vi "UItoDAQconfig.vi"(8 "SamplingInfo":cluster{"Fs":dbl, "#S":i32}={"Fs"=1000.0, "#S"=1000}, 9 "AO Configuration":T7, 10 "AI Configuration":T10, 11 "DAQ_Manager.setDAQConfig":T1 {"DAQmx.AI.config"."input terminal configuration" items=["default"=-1, "RSE"=10083, "NRSE"=10078, "Differential"=10106, "Pseudodifferential"=12529]; "DAQmx.AI.config"."AI.Coupling" items=["AC"=10045, "DC"=10050, "GND"=10066]; "DAQmx.AO.config"."output terminal configuration" items=["Default"=-1, "RSE"=10083, "Differential"=10106, "Pseudodifferential"=12529]}) -> (3 "DAQ_Manager.setDAQConfig":T1 {"DAQmx.AI.config"."input terminal configuration" items=["default"=-1, "RSE"=10083, "NRSE"=10078, "Differential"=10106, "Pseudodifferential"=12529]; "DAQmx.AI.config"."AI.Coupling" items=["AC"=10045, "DC"=10050, "GND"=10066]; "DAQmx.AO.config"."output terminal configuration" items=["Default"=-1, "RSE"=10083, "Differential"=10106, "Pseudodifferential"=12529]})   [LabVIEW 2019, in "UI.Lockin.DAQ_config.lvclass"]
uses:
  UI.Lockin.DAQ_config.lvclass
  Typedefs/AI.config-array.ctl
  Typedefs/AI.config-cluster.ctl
  Typedefs/AI.coupling-enum.ctl
  Typedefs/446xAI-enum.ctl
  Typedefs/AO.config-array.ctl
  Typedefs/AO.config-cluster.ctl
  Typedefs/446xAO-enum.ctl
  DAQ_Manager/Typedefs/PrivateEvents--DAQ_Manager.setDAQConfig.ctl
  DAQmx.AI/Typedefs/DAQmx.AI_Config.ctl
  DAQmx.AI/Typedefs/AI.Coupling-enum.ctl
  DAQmx.AI/Typedefs/AI.Terminal-enum.ctl
  DAQmx.AO/Typedefs/DAQmx.AO_Config.ctl
  DAQmx.AO/Typedefs/AO.Terminal-enum.ctl
  DAQmx.AI/DAQmx.AI.lvclass
  DAQmx.AO/DAQmx.AO.lvclass
  DAQ_Manager/DAQ_Manager.lvclass
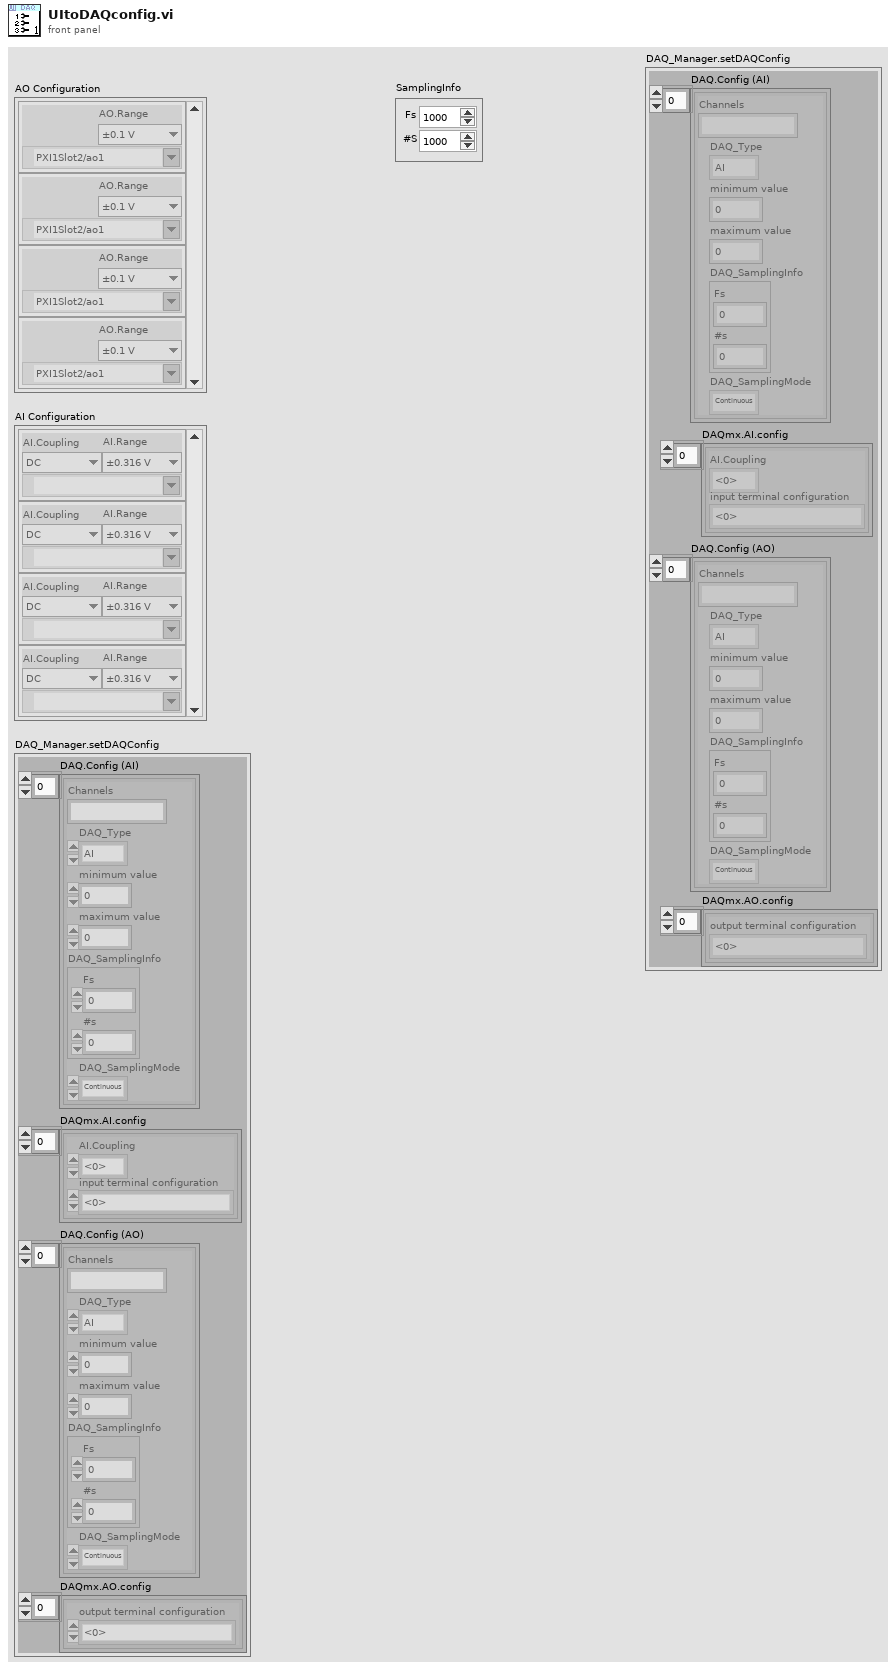
[diagram p1: front panel]
types:
  T1 = typedef "DAQ_Manager.lvclass/PrivateEvents--DAQ_Manager.setDAQConfig.ctl" = cluster{"DAQ.Config (AI)":cluster{"Channels":string, "DAQ_Type":enum16{"AI", "AO"}, "minimum value":dbl, "maximum value":dbl, "DAQ_SamplingInfo":cluster{"Fs":dbl, "#s":i32}, "DAQ_SamplingMode":enum16{"Continuous", "Finite"}}[], "DAQmx.AI.config":T2[], "DAQ.Config (AO)":cluster{"Channels":string, "DAQ_Type":enum16{"AI", "AO"}, "minimum value":dbl, "maximum value":dbl, "DAQ_SamplingInfo":cluster{"Fs":dbl, "#s":i32}, "DAQ_SamplingMode":enum16{"Continuous", "Finite"}}[], "DAQmx.AO.config":T5[]}
  T2 = typedef "DAQmx.AI.lvclass/DAQmx.AI_Config.ctl" = cluster{"AI.Coupling":T3, "input terminal configuration ":T4}
  T3 = typedef "DAQmx.AI.lvclass/AI.Coupling-enum.ctl" = i32
  T4 = typedef "DAQmx.AI.lvclass/AI.Terminal-enum.ctl" = i32
  T5 = typedef "DAQmx.AO.lvclass/DAQmx.AO_Config.ctl" = cluster{"output terminal configuration":T6}
  T6 = typedef "DAQmx.AO.lvclass/AO.Terminal-enum.ctl" = i32
  T7 = typedef "UI.Lockin.DAQ_config.lvclass/AO.config-array.ctl" = T8[]
  T8 = typedef "UI.Lockin.DAQ_config.lvclass/AO.config-cluster.ctl" = cluster{"AO.Range":T9, "DAQmx Physical Channel":tag}
  T9 = typedef "UI.Lockin.DAQ_config.lvclass/446xAO-enum.ctl" = enum16{"±0.1 V", "±1.0 V", "±10.0 V"}
  T10 = typedef "UI.Lockin.DAQ_config.lvclass/AI.config-array.ctl" = T11[]
  T11 = typedef "UI.Lockin.DAQ_config.lvclass/AI.config-cluster.ctl" = cluster{"AI.Coupling":T12, "AI.Range":T13, "DAQmx Physical Channel":tag}
  T12 = typedef "UI.Lockin.DAQ_config.lvclass/AI.coupling-enum.ctl" = enum16{"AC", "DC"}
  T13 = typedef "UI.Lockin.DAQ_config.lvclass/446xAI-enum.ctl" = enum16{"±0.316 V", "±1.00 V", "±3.16 V", "±10.0 V", "±31.6 V", "±42.4 V"}
  T14 = cluster{"Channels":string, "DAQ_Type":enum16{"AI", "AO"}, "minimum value":dbl, "maximum value":dbl, "DAQ_SamplingInfo":cluster{"Fs":dbl, "#s":i32}, "DAQ_SamplingMode":enum16{"Continuous", "Finite"}}[]
  T15 = cluster{"Channels":string, "DAQ_Type":enum16{"AI", "AO"}, "minimum value":dbl, "maximum value":dbl, "DAQ_SamplingInfo":cluster{"Fs":dbl, "#s":i32}, "DAQ_SamplingMode":enum16{"Continuous", "Finite"}}
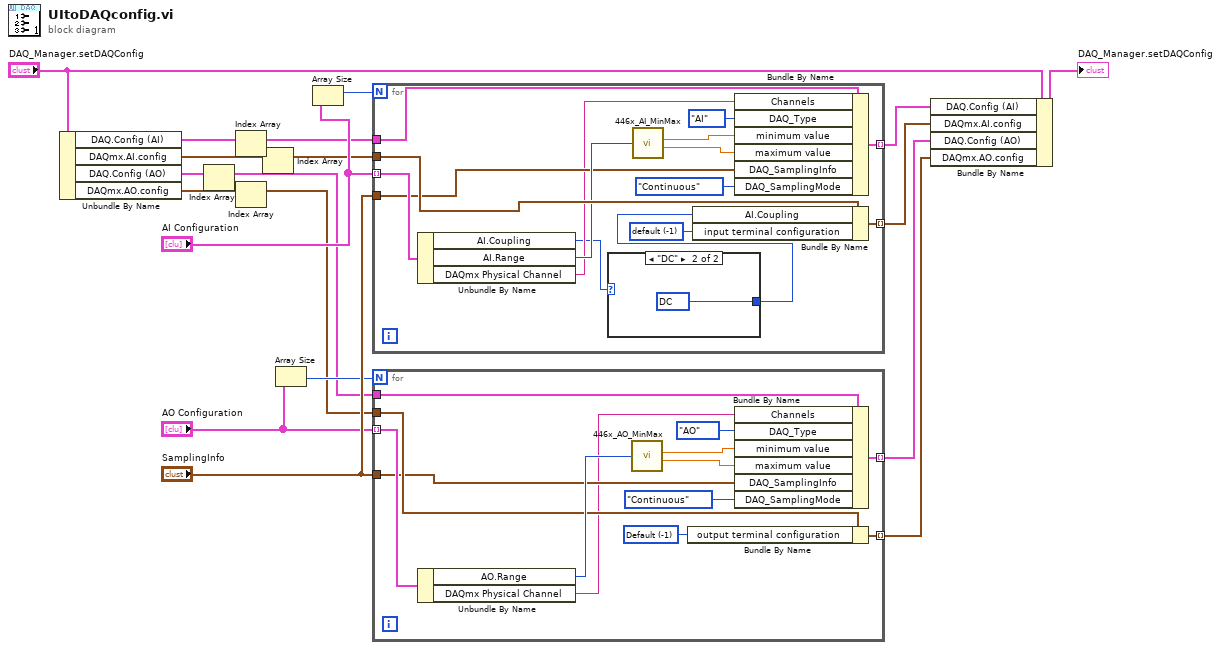
[diagram p0: block diagram]
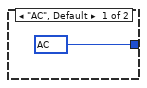
[diagram p2: hidden frame]
diagram:
  n1 = Unbundle By Name("DAQ_Manager.setDAQConfig") -> ("DAQ.Config (AI)"=w16:T14, "DAQmx.AI.config"=w17:T2[], "DAQ.Config (AO)"=w18:T14, "DAQmx.AO.config"=w19:T5[])
  n2 = Index Array(array=w18) -> (element=w1:T15)  [unwired: 1 in]
  n3 = Index Array(array=w16) -> (element=w4:T15)  [unwired: 1 in]
  n4 = Index Array(array=w19) -> (element=w2:T5)  [unwired: 1 in]
  n5 = Index Array(array=w17) -> (element=w3:T2)  [unwired: 1 in]
  n6 = Array Size(array="AO Configuration") -> (size(s)=w7:i32)
  n7 = Array Size(array="AI Configuration") -> (size(s)=w5:i32)
  n8 = for {
    N: w5 -> [_]
    tunnel: w4 -> [w33]
    tunnel: w3 -> [w32]
    tunnel: "AI Configuration" -> [w34] mode=indexing
    tunnel: "SamplingInfo" -> [w27]
    tunnel: [w23] -> w12 mode=indexing
    tunnel: [w22] -> w11 mode=indexing
    w29 = T4 -1 items=["default"=-1, "RSE"=10083, "NRSE"=10078, "Differential"=10106, "Pseudodifferential"=12529] ("input terminal configuration")
    n9 = Unbundle By Name(w34) -> ("AI.Coupling"=w21:T12, "AI.Range"=w30:T13, "DAQmx Physical Channel"=w25:tag)
    n10 = case shown="\"DC\"" w21 {
      tunnel: [w35 w36] -> w20
      frame "AC", Default {
        w35 = T3 10045 items=["AC"=10045, "DC"=10050, "GND"=10066] ("AI.Coupling")
      }
      frame "DC" {
        w36 = T3 10050 items=["AC"=10045, "DC"=10050, "GND"=10066] ("AI.Coupling")
      }
    }
    n11 = call "446x_AI_MinMax.vi"("446x AI"=w30) -> ("AI.Min"=w31:dbl, "AI.Max"=w24:dbl)  [unwired: 6 in]
    n12 = Bundle By Name(cluster=w32, "AI.Coupling"=w20, "input terminal configuration"=w29) -> (w22:T2)
    n13 = Bundle By Name(cluster=w33, "Channels"=w25, "DAQ_Type"=enum16{"AI", "AO"}."AI", "minimum value"=w31, "maximum value"=w24, "DAQ_SamplingInfo"=w27, "DAQ_SamplingMode"=enum16{"Continuous", "Finite"}."Continuous") -> (w23:T15)
  }
  n14 = for {
    N: w7 -> [_]
    tunnel: w1 -> [w47]
    tunnel: w2 -> [w46]
    tunnel: "AO Configuration" -> [w49] mode=indexing
    tunnel: "SamplingInfo" -> [w43]
    tunnel: [w38] -> w10 mode=indexing
    tunnel: [w37] -> w9 mode=indexing
    w45 = T6 -1 items=["Default"=-1, "RSE"=10083, "Differential"=10106, "Pseudodifferential"=12529] ("output terminal configuration")
    n15 = Unbundle By Name(w49) -> ("AO.Range"=w48:T9, "DAQmx Physical Channel"=w39:tag)
    n16 = call "446x_AO_MinMax.vi"("AO.Range"=w48) -> ("AO.min"=w41:dbl, "AO.max"=w40:dbl)  [unwired: 6 in]
    n17 = Bundle By Name(cluster=w46, "output terminal configuration"=w45) -> (w37:T5)
    n18 = Bundle By Name(cluster=w47, "Channels"=w39, "DAQ_Type"=enum16{"AI", "AO"}."AO", "minimum value"=w41, "maximum value"=w40, "DAQ_SamplingInfo"=w43, "DAQ_SamplingMode"=enum16{"Continuous", "Finite"}."Continuous") -> (w38:T15)
  }
  n19 = Bundle By Name(cluster="DAQ_Manager.setDAQConfig", "DAQ.Config (AI)"=w12, "DAQmx.AI.config"=w11, "DAQ.Config (AO)"=w10, "DAQmx.AO.config"=w9) -> (→"DAQ_Manager.setDAQConfig":T1)
